vi "LiquidFlowIn.vi"(9 "level_increase_in_points":i32, 10 "room_temperature":dbl, 11 "liquid_temperature":dbl[][](array[numeric])) -> (3 "new_liquid_temperature":dbl[][](array[numeric]))   [LabVIEW 2020]
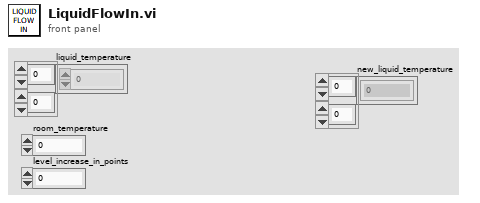
[diagram p1: front panel]
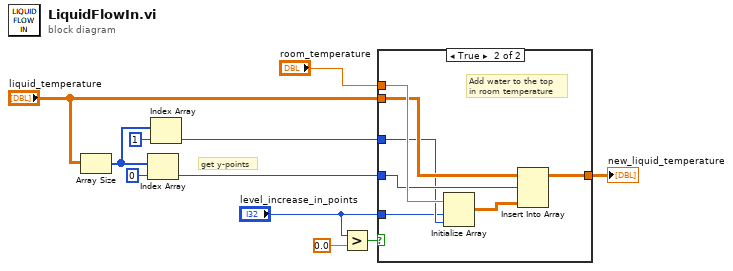
[diagram p0: block diagram]
diagram:
  # "get y-points"
  n1 = Array Size(array="liquid_temperature") -> (size(s)=w8:i32[])
  n2 = Index Array(array=w8, index=0) -> (element=w10:i32)
  n3 = Index Array(array=w8, index=1) -> (element=w7:i32)
  n4 = Greater?(x="level_increase_in_points", y=0.0) -> (0:w6:bool)
  n5 = case shown="True" w6 {
    tunnel: "liquid_temperature" -> [w12 w18]
    tunnel: [w12 w17] -> w3
    tunnel: w10 -> [_ w16]
    tunnel: "room_temperature" -> [_ w19]
    tunnel: w7 -> [_ w15]
    tunnel: "level_increase_in_points" -> [_ w13]
    frame False {
    }
    frame True {
      # "Add water to the top\nin room temperature"
      n6 = Initialize Array(w19, w13, w15) -> (w14:dbl[][])
      n7 = Insert Into Array(array=w18, index (row)=w16, new element=w14) -> (w17:dbl[][])  [unwired: 1 in]
    }
  }
  "new_liquid_temperature" <- w3
